vi "Add Blueprint.vi"(8 "error in (no error)":errorcluster, 10 "Blueprint":refnum<class "Blueprint.lvclass">, 11 "App in":refnum<class "App.lvclass">) -> (0 "error out":errorcluster, 3 "App out":refnum<class "App.lvclass">)   [LabVIEW 2020, in "App.lvclass"]
uses:
  App.lvclass
  Blueprint/Blueprint.lvclass
  Blueprint Qty.ctl
  App.lvclass/App.ctl
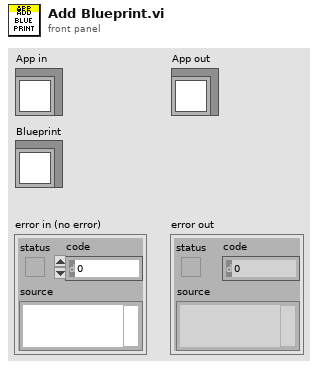
[diagram p1: front panel]
types:
  T1 = typedef "App.lvclass/Blueprint Qty.ctl" = cluster{"Blueprint":refnum<class "Blueprint.lvclass">, "Qty":dbl}
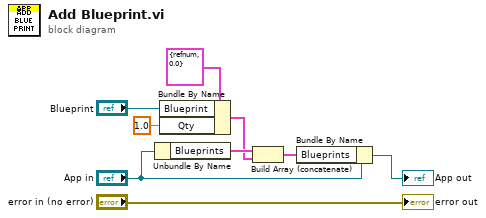
[diagram p0: block diagram]
diagram:
  n1 = Unbundle By Name("App in") -> ("Blueprints"=w8:T1[])
  n2 = Bundle By Name(cluster=T1 {"Blueprint"=refnum, "Qty"=0.0} ("Blueprint Qty"), "Blueprint"="Blueprint", "Qty"=1.0) -> (w4:T1)
  n3 = Build Array (concatenate)(w8, w4) -> (w3:T1[])
  n4 = Bundle By Name(cluster="App in", "Blueprints"=w3) -> (→"App out":refnum<class "App.lvclass">)
  "error out" <- "error in (no error)"
